vi "Restore Permissions.vi"(8 "Error In":errorcluster, 11 "File Path":path) -> (0 "Error Out":errorcluster, 3 "Duplicate File Path":path)   [LabVIEW 2016]
panel:
  out "return code":i32
  out "standard error":string
  out "standard output":string
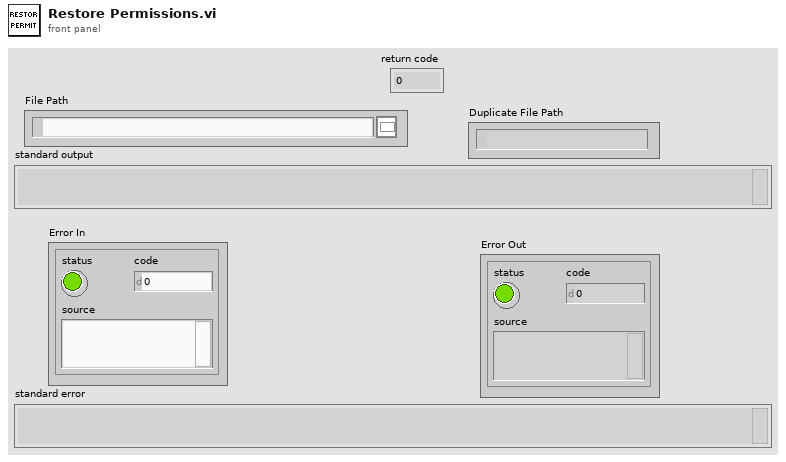
[diagram p1: front panel]
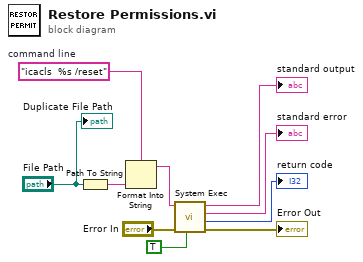
[diagram p0: block diagram]
diagram:
  w10 = "icacls  %s /reset"  # command line
  n1 = Path To String(path="File Path") -> (string=w9:string)
  n2 = Format Into String(format string=w10, w9) -> (resulting string=w8:string)  [unwired: 2 in, 1 out]
  n3 = call <vilib>:"System Exec.vi"("run minimized? (F)"=TRUE, "error in (no error)"="Error In", "command line"=w8) -> ("error out"=→"Error Out":errorcluster, "return code"=→"return code":i32, "standard error"=→"standard error":string, "standard output"=→"standard output":string)  [unwired: 3 in, 2 out]
  "Duplicate File Path" <- "File Path"
